vi "Untitled 3 (SubVI).vi"(6 "disabled index (col)":i32, 9 "index (row)":i32, 10 "Velocity Component 2 Out":T1, 11 "Refnum in":T1) -> (3 "appended array":sgl[](array[numeric]))   [LabVIEW 2014]
uses:
  <vilib>/vision/Image Controls.llb/IMAQ Image.ctl
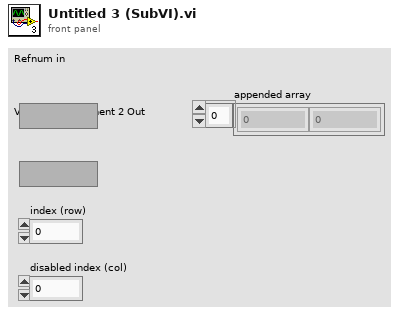
[diagram p1: front panel]
types:
  T1 = typedef "IMAQ Image.ctl" = refnum<image>
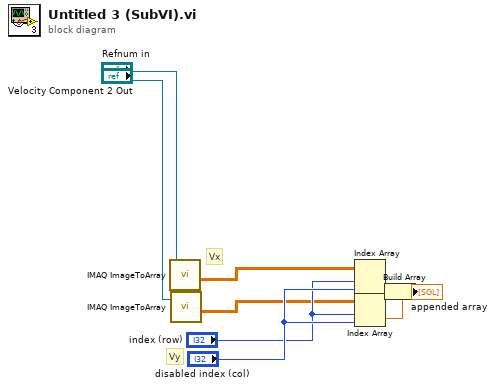
[diagram p0: block diagram]
diagram:
  # "Vy"
  # "Vx"
  n1 = call "IMAQ ImageToArray"("Image"="Refnum in") -> ("Image Pixels (Float)"=w3:sgl[][])  [unwired: 3 in, 4 out]
  n2 = call "IMAQ ImageToArray"("Image"="Velocity Component 2 Out") -> ("Image Pixels (Float)"=w4:sgl[][])  [unwired: 3 in, 4 out]
  n3 = Index Array(array=w3, index (row)="index (row)", index (col)="disabled index (col)") -> (element=w7:sgl)
  n4 = Index Array(array=w4, index (row)="index (row)", index (col)="disabled index (col)") -> (element=w8:sgl)
  n5 = Build Array(w7, w8) -> (→"appended array":sgl[])
